vi "Get View Status.vi"(8 "error in (no error)":errorcluster, 10 "View":string, 11 "GUI Container View Actor in":refnum<class "GUI Container Actor.lvclass">) -> (0 "error out":errorcluster, 1 "View Found":bool, 2 "View Status":T1, 3 "GUI Container View Actor out":refnum<class "GUI Container Actor.lvclass">)   [LabVIEW 2023, in "GUI Views.lvlib" / "GUI Container Actor.lvclass"]
uses:
  GUI Container Actor.lvclass
  typedefs/View Status.ctl
  <vilib>/ActorFramework/Message Enqueuer/Message Enqueuer.lvclass
  typedefs/View Details.ctl
  typedefs/FP Status.ctl
  GUI Container Actor.lvclass/GUI Container Actor.ctl
  <userlib>/_OpenG.lib/error/error.llb/openg_error.lvlib
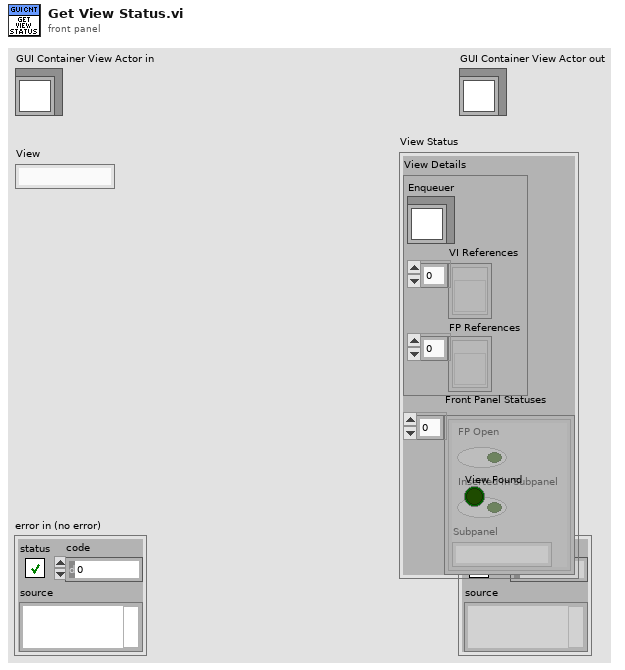
[diagram p1: front panel]
types:
  T1 = typedef "GUI Views.lvlib/GUI Container Actor.lvclass/View Status.ctl" = cluster{"View Details":T2, "Front Panel Statuses":T3[]}
  T2 = typedef "GUI Views.lvlib/GUI Container Actor.lvclass/View Details.ctl" = cluster{"Enqueuer":refnum<class "Message Enqueuer.lvclass">, "VI References":refnum<vi>[], "FP References":refnum<vi>[]}
  T3 = typedef "GUI Views.lvlib/GUI Container Actor.lvclass/FP Status.ctl" = cluster{"FP Open":bool, "Inserted in Subpanel":bool, "Subpanel":string}
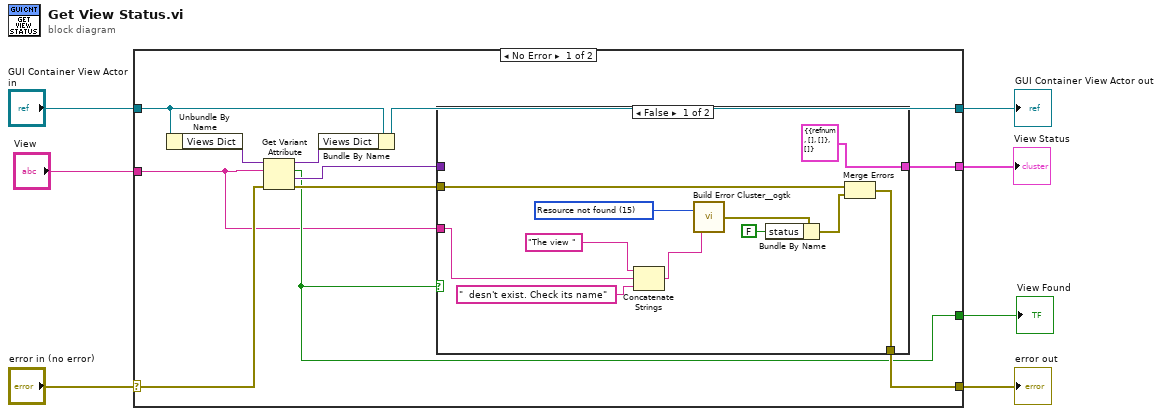
[diagram p0: block diagram]
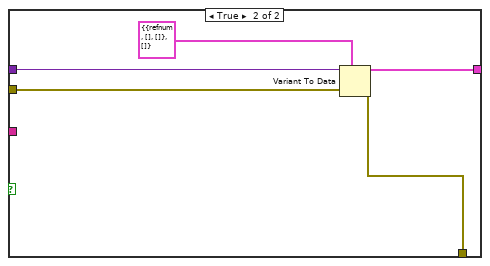
[diagram p2: hidden frame]
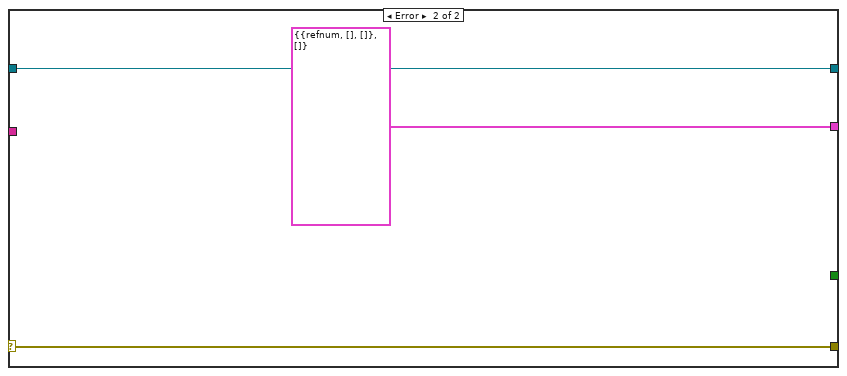
[diagram p3: hidden frame]
diagram:
  n1 = case shown="No Error" "error in (no error)" {
    selector: "error in (no error)" -> [w16 w37]
    tunnel: [w10 w37] -> w6
    tunnel: [w15 w36] -> w4
    tunnel: "GUI Container View Actor in" -> [w18 w36]
    tunnel: "View" -> [w8 _]
    tunnel: [w11 T1 {"View Details"={"Enqueuer"=refnum, "VI References"=[], "FP References"=[]}, "Front Panel Statuses"=[]} ("View State")] -> w2
    tunnel: [w9 _] -> w1
    frame No Error {
      n2 = Unbundle By Name(w18) -> ("Views Dict"=w17:variant)
      n3 = Get Variant Attribute(Variant=w17, name=w8, error in=w16) -> (duplicate Variant=w14:variant, found=w9:bool, value=w12:variant, error out=w13:errorcluster)  [unwired: 1 in]
      n4 = Bundle By Name(cluster=w18, "Views Dict"=w14) -> (w15:refnum<class "GUI Container Actor.lvclass">)
      n5 = case shown="False" w9 {
        tunnel: w13 -> [w24 w34]
        tunnel: w12 -> [_ w33]
        tunnel: [T1 {"View Details"={"Enqueuer"=refnum, "VI References"=[], "FP References"=[]}, "Front Panel Statuses"=[]} ("View State") w31] -> w11
        tunnel: [w23 w30] -> w10
        tunnel: w8 -> [w22 _]
        frame False {
          w25 = 15 items=["No error", "Argument error", "Memory is full", "Out of zone", "End of file", "File already open", "Generic file I/O error", "File not found", "File permission error", "Disk is full", "Duplicate path", "Too many files open", "System feature not enabled", "Resource file not found", "Cannot add resource", "Resource not found", "Image not found", "Image memory error", "Pen does not exist", "Config type invalid", "Config token not found", "Config parse error", "Config memory error", "Bad external code format", "Bad external code offset", "External code not present", "Null window", "Destroy window error", "Null menu", "Print aborted", "Bad print record", "Print driver error", "Windows error during printing", "Memory error during printing", "Print dialog error", "Generic print error", "Invalid device refnum", "Device not found", "Device parameter error", "Device unit error", "Cannot open device", "Device call aborted", "Generic error", "Cancelled by user", "Object ID too low", "Object ID too high", "Object not in heap", "Unknown heap", "Unknown object (invalid DefProc)", "Unknown object (DefProc not in table)", "Message out of range", "Invalid (null) method", "Unknown message", "Manager call not supported", "Bad address", "Network operation in progress", "Network operation timed out", "Connection is busy", "Network attribute not supported", "Network error", "Address in use", "System out of memory", "Connection aborted", "Connection refused", "Not connected", "Already connected", "Connection closed", "Initialization error (interapplication manager)", "Bad occurrence", "Wait on unbound occurrence handler", "Occurrence queue overflow", "Datalog type conflict", "Unused", "Unrecognized type (interapplication manager)", "Memory corrupt", "Failed to make temporary DLL", "Old CIN version", "Drag socket not found", "Failed to load drop-object", "Failed to register OLE object", "Failed to release OLE object", "Format specifier type mismatch", "Unknown format specifier", "Too few format specifiers", "Too many format specifiers", "Scan failed", "Newer CIN version", "Error converting to variant", "Runtime menu error", "Password tampered", "Variant attribute not found", "Incompatible variant data type", "Event data is not available", "Event Store is not present", "Occurrence is not found", "Event Queue is not created", "Event info is not available", "Refnum passed is NULL", "Error retrieving Class GUID", "Error retrieving CoClass GUID", "Error retrieving TypeLib GUID.", "Bad built application magic bytes.", "Specific driver is different from the specific driver associated with the Logical Name.", "There is no session opened to the class driver.", "Max Error", "MAX - Error with config objects", "MAX - Error loading configuration", "MAX - Group not supported"]
          n6 = Concatenate Strings("The view " ("String to Prepend to source (\"\")"), w22, "  desn't exist. Check its name" ("string")) -> (w28:string)
          n7 = call <userlib>:"Build Error Cluster__ogtk.vi"("String to Prepend to source (\"\")"=w28, "code"=w25) -> ("error out"=w29:errorcluster)
          n8 = Bundle By Name(cluster=w29, "status"=FALSE) -> (w20:errorcluster)
          n9 = Merge Errors(w24, w20) -> (w23:errorcluster)
        }
        frame True {
          n10 = Variant To Data(error in=w34, type=T1 {"View Details"={"Enqueuer"=refnum, "VI References"=[], "FP References"=[]}, "Front Panel Statuses"=[]} ("View State"), Variant=w33) -> (data=w31:T1, error out=w30:errorcluster)
        }
      }
    }
    frame Error {
    }
  }
  "error out" <- w6
  "GUI Container View Actor out" <- w4
  "View Status" <- w2
  "View Found" <- w1
